vi "read_dust_control_settings_small.vi"(7 "Settings to be loaded":i32, 8 "error in (no error)":errorcluster, 9 "Tag Filter":cluster{"Tag":string, "Dust Type":string}, 10 "Lower Timestamp Range":timestamp, 11 "Upper Timestamp Range":timestamp) -> (0 "error out":errorcluster, 1 "Array":cluster{"String":string, "Value":dbl}[](array[cluster]), 3 "Dust Source Array":T1[](array[typedef]) {"Needle Voltage" min=0.0 max=10.0 step=0.01 format="%.2g"; "Desired Amplitude (V)" min=0.0 max=10.0 step=0.01 format="%5.2f"; "Width (ms) : 0.1" min=0.05 max=5.0 step=0.01 format="%6.2f"; "Frequency" min=1.0 max=100.0 step=0.01 format="%.1f"})   [LabVIEW 2013]
uses:
  dust_source_control_small.ctl
  <vilib>/addons/database/Auxilliary.llb/DB Tools Cursor Type.ctl
  <vilib>/addons/database/Connection.llb/Conn Execute.vi
  <vilib>/addons/database/Recordset.llb/Rec Fetch Recordset Data (R).vi
  <vilib>/addons/database/Recordset.llb/Rec Destroy - Connection.vi
  <vilib>/addons/database/_DB Variant To Data/Database Variant To Data.xnode
  <vilib>/addons/database/NI_Database_API.lvlib
panel:
  out "Settings ID 2":dbl(ring) caption="Settings ID" items=["Auto", "Auto", "Auto", "Auto", "Auto", "Auto", "Auto", "Auto", "Auto", "Auto", "Auto", "Auto", "Auto", "Auto", "Auto", "Auto", "Auto", "Auto", "Auto", "Auto", "Auto test", "Auto", "Automatic Update at  10/19/2012 4:35:52 PM", "Automatic Update at  10/19/2012 4:37:24 PM", "Automatic Update at  10/19/2012 4:37:56 PM", "Automatic Update at  10/19/2012 4:39:59 PM", "Automatic Update at  10/19/2012 4:40:46 PM", "Automatic Update at  10/19/2012 4:43:56 PM", "Automatic Update at  10/19/2012 5:03:34 PM", "Awesome settings that work", "Awesome settings that work", "Automatic Update at  10/19/2012 5:32:08 PM", "Automatic Update at  10/19/2012 5:34:15 PM", "Automatic Update at  10/19/2012 5:39:51 PM", "Working settings", "Working settings", "Working settings", "Working settings", "Working settings", "Automatic Update at  10/22/2012 1:18:52 PM", "Automatic Update at  10/22/2012 1:22:32 PM", "", "Test", "Test", "Automatic Update at  10/22/2012 1:29:56 PM", "Test", "Test 1", "Test 1", "Anna's Settings", "Automatic Update at  10/22/2012 3:57:19 PM", "test of width", "Automatic Update at  10/22/2012 4:02:00 PM", "Automatic Update at  10/22/2012 4:10:30 PM", "Automatic Update at  10/22/2012 4:15:00 PM", "Automatic Update at  10/22/2012 4:38:33 PM", "Automatic Update at  10/22/2012 4:44:48 PM", "Automatic Update at  10/22/2012 4:46:11 PM", "Automatic Update at  10/22/2012 4:51:36 PM", "Automatic Update at  10/22/2012 4:54:36 PM", "Automatic Update at  10/22/2012 4:59:09 PM", "Automatic Update at  10/22/2012 5:01:02 PM", "Automatic Update at  10/22/2012 5:06:29 PM", "Automatic Update at  10/22/2012 5:13:46 PM", "Automatic Update at  10/22/2012 5:18:54 PM", "Automatic Update at  10/22/2012 5:27:58 PM", "Automatic Update at  10/22/2012 5:37:45 PM", "Automatic Update at  10/22/2012 5:39:44 PM", "Automatic Update at  10/22/2012 5:41:21 PM", "Automatic Update at  10/22/2012 5:41:55 PM", "Automatic Update at  10/22/2012 5:43:41 PM", "Automatic Update at  10/22/2012 5:45:31 PM", "Anna's Settings (Updated with working Giraffes)", "Anna's Settings (Updated with working Giraffes)", "Automatic Update at  10/23/2012 1:01:38 PM", "test", "test", "test 1", "test 1", "Automatic Update at  10/23/2012 1:44:56 PM", "Automatic Update at  10/23/2012 1:52:29 PM", "Automatic Update at  10/23/2012 1:59:24 PM", "test 3", "test 4", "Automatic Update at  10/23/2012 2:20:20 PM", "Automatic Update at  10/23/2012 5:53:49 PM", "Anna's Settings", "Anna's Settings1", "test mctesty", "test mctesty", "Automatic Update at  10/24/2012 3:47:44 PM", "Test\"", "Test\"", "this is a \"test\" setting", "Automatic Update at  10/24/2012 4:13:56 PM"]
  out "SQL Query Sintax":string
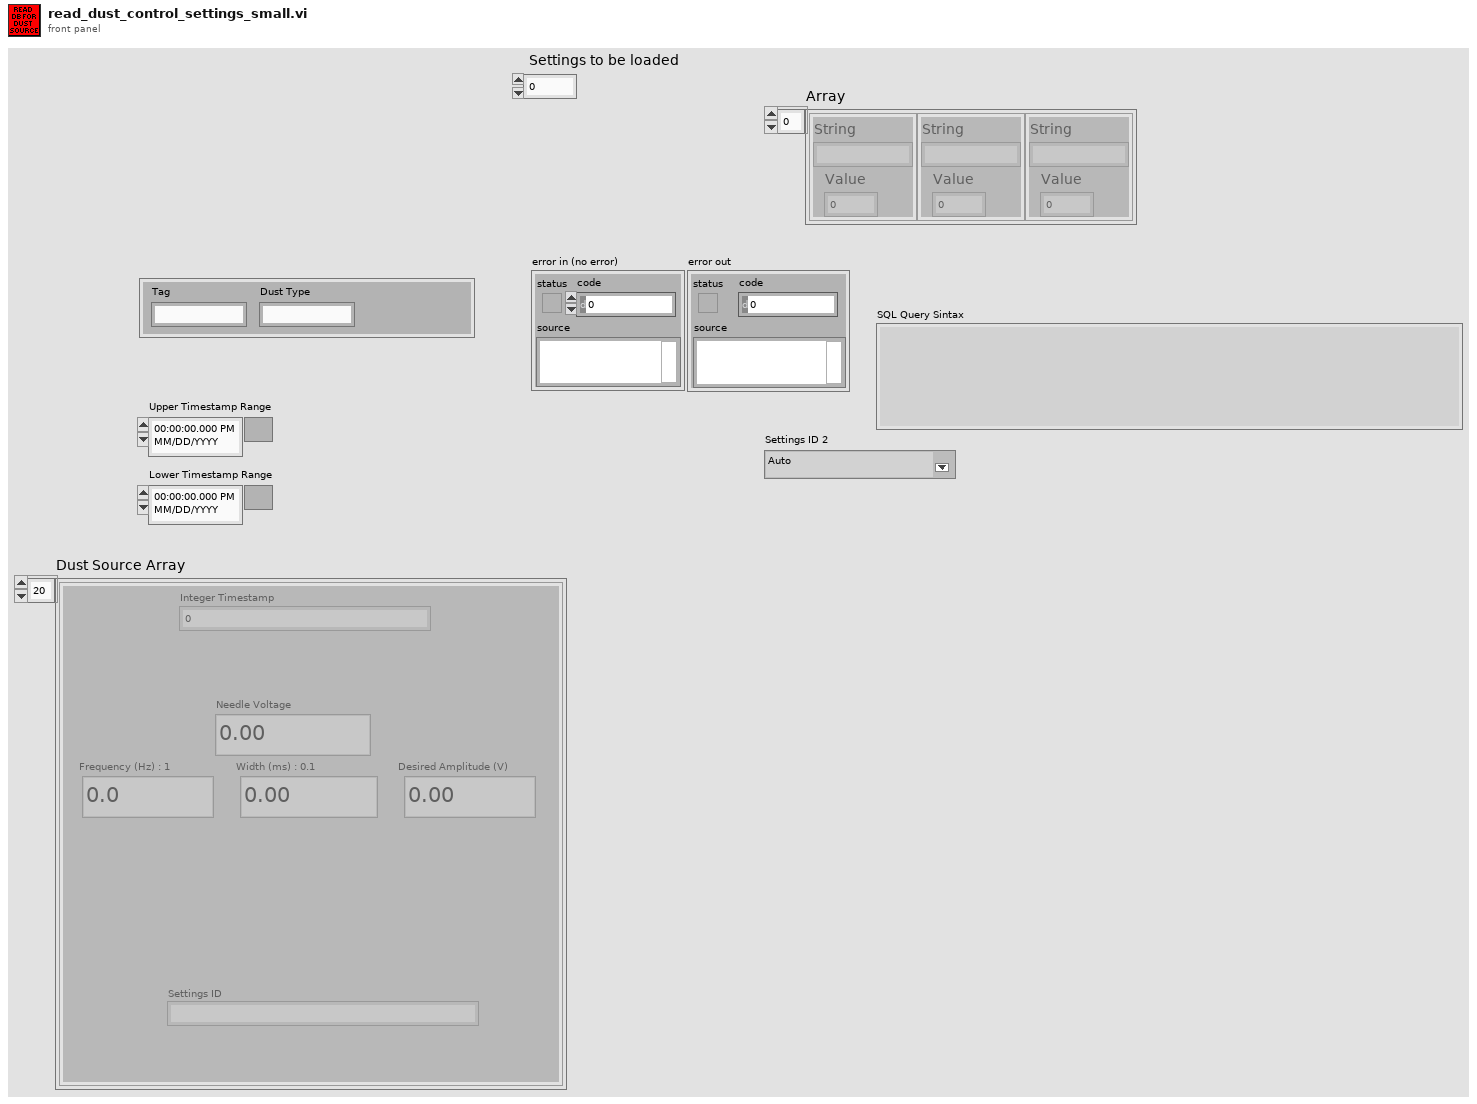
[diagram p1: front panel]
types:
  T1 = typedef "dust_source_control_small.ctl" = cluster{"Integer Timestamp":u64, "Needle Voltage":dbl, "Frequency":dbl, "Width (ms) : 0.1 ":dbl, "Desired Amplitude (V)":dbl, "Settings ID":string, "ID#":i32}
  T2 = typedef "NI_Database_API.lvlib/DB Tools Cursor Type.ctl" = enum16{"forward-only", "keyset", "dynamic", "static"}
  T3 = typedef "NI_Database_API.lvlib/Conn ObjectReference.ctl" = refnum<k1>
  T4 = typedef "NI_Database_API.lvlib/Rec ObjectReference.ctl" = refnum<k1>
  T5 = cluster{"Integer Timestamp":u64, "Needle Voltage":dbl, "Frequency":dbl, "Width (ms) : 0.1 ":dbl, "Desired Amplitude (V)":dbl, "Settings ID":string, "ID#":i32}
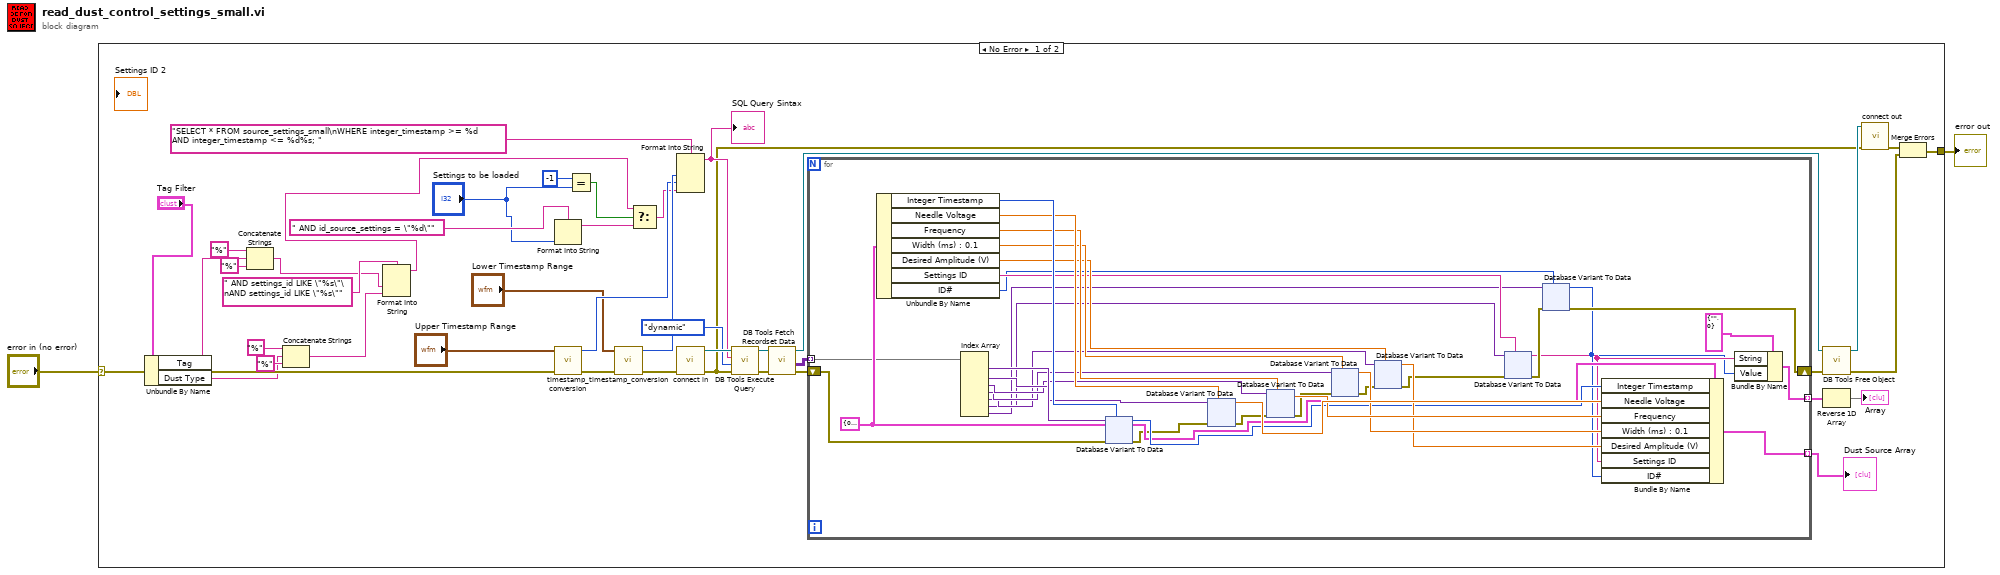
[diagram p0: block diagram]
diagram:
  n1 = case shown="No Error" "error in (no error)" {
    selector: "error in (no error)" -> [w35 w303]
    tunnel: [w19 w303] -> w1
    frame No Error {
      n2 = Unbundle By Name("Tag Filter") -> ("Tag"=w9:string, "Dust Type"=w7:string)
      n3 = Concatenate Strings("%" ("string"), w9, "%" ("string")) -> (w10:string)
      n4 = Concatenate Strings("%" ("string"), w7, "%" ("string")) -> (w5:string)
      n5 = Format Into String(format string=" AND settings_id LIKE \"%s\"\nAND settings_id LIKE \"%s\"" ("string"), w10, w5) -> (resulting string=w4:string)  [unwired: 2 in, 1 out]
      n6 = Format Into String(format string=" AND id_source_settings = \"%d\"" ("string"), "Settings to be loaded") -> (resulting string=w31:string)  [unwired: 2 in, 1 out]
      n7 = call "timestamp_conversion.vi"("error in (no error)"=w35, "Time Stamp"="Upper Timestamp Range") -> ("error out"=w36:errorcluster, "Integer Time"=w29:i64)  [unwired: 7 in]
      n8 = Equal?(x=-1, y="Settings to be loaded") -> (x = y?=w37:bool)
      n9 = call "timestamp_conversion.vi"("error in (no error)"=w36, "Time Stamp"="Lower Timestamp Range") -> ("error out"=w33:errorcluster, "Integer Time"=w30:i64)  [unwired: 7 in]
      n10 = Select(t=w4, s=w37, f=w31) -> (s? t:f=w23:string)
      n11 = Format Into String(format string="SELECT * FROM source_settings_small\nWHERE integer_timestamp >= %d  AND integer_timestamp <= %d%s; " ("string"), w30, w29, w23) -> (resulting string=w27:string)  [unwired: 2 in, 1 out]
      "SQL Query Sintax" <- w27
      n12 = call "connect in.vi"("error in (no error)"=w33) -> ("error out"=w17:errorcluster, "Database Connection"=w39:T3)  [unwired: 6 in, 1 out]
      n13 = call-poly <vilib>:"DB Tools Execute Query.vi"("error in (no error)"=w17, "cursor type"=DB_Tools_Cursor_Type."dynamic", "SQL query"=w27, "connection reference"=w39) -> ("error out"=w43:errorcluster, "recordset reference"=w44:T4)  [unwired: 4 in]
      n14 = call-poly <vilib>:"DB Tools Fetch Recordset Data.vi"("error in (no error)"=w43, "recordset reference"=w44) -> ("error out"=w41:errorcluster, "recordset data"=w34:variant[][], "recordset reference out"=w42:T4)  [unwired: 3 in]
      n15 = for {
        tunnel: w34 -> [w67] mode=indexing
        shift-right: [w58] -> w40
        shift-left: w41 -> [w78]
        tunnel: [w70] -> w14 mode=indexing
        tunnel: [w55] -> w22 mode=indexing
        w68 = T5 {"Integer Timestamp"=0, "Needle Voltage"=0.0, "Frequency"=1.0, "Width (ms) : 0.1 "=0.05, "Desired Amplitude (V)"=0.0, "Settings ID"="", "ID#"=0} ("Dust Source Controls")
        n16 = Unbundle By Name(w68) -> ("Integer Timestamp"=w66:u64, "Needle Voltage"=w64:dbl, "Frequency"=w63:dbl, "Width (ms) : 0.1"=w62:dbl, "Desired Amplitude (V)"=w61:dbl, "Settings ID"=w60:string, "ID#"=w57:i32)
        n17 = Index Array(array=w67) -> (element #1=w65:variant, element #2=w50:variant, element #3=w49:variant, element #4=w48:variant, element #5=w47:variant, element #6=w46:variant, element #7=w45:variant)  [unwired: 7 in]
        n18 = xnode "Database Variant To Data"("database variant"=w65, "error in"=w78, "type"=w66) -> ("data"=w69:u64, "error out"=w52:errorcluster)
        n19 = xnode "Database Variant To Data"("database variant"=w50, "error in"=w52, "type"=w64) -> ("data"=w77:dbl, "error out"=w75:errorcluster)
        n20 = xnode "Database Variant To Data"("database variant"=w49, "error in"=w75, "type"=w63) -> ("data"=w76:dbl, "error out"=w73:errorcluster)
        n21 = xnode "Database Variant To Data"("database variant"=w48, "error in"=w73, "type"=w62) -> ("data"=w74:dbl, "error out"=w72:errorcluster)
        n22 = xnode "Database Variant To Data"("database variant"=w47, "error in"=w72, "type"=w61) -> ("data"=w71:dbl, "error out"=w51:errorcluster)
        n23 = xnode "Database Variant To Data"("database variant"=w46, "error in"=w51, "type"=w60) -> ("data"=w54:string, "error out"=w59:errorcluster)
        n24 = xnode "Database Variant To Data"("database variant"=w45, "error in (no error)"=w59, "type"=w57) -> ("data"=w53:i32, "error out"=w58:errorcluster)
        n25 = Bundle By Name(cluster=w68, "Integer Timestamp"=w69, "Needle Voltage"=w77, "Frequency"=w76, "Width (ms) : 0.1"=w74, "Desired Amplitude (V)"=w71, "Settings ID"=w54, "ID#"=w53) -> (w70:T5)
        n26 = Bundle By Name(cluster=cluster{"String":string, "Value":i32} {"String"="", "Value"=0}, "String"=w54, "Value"=w53) -> (w55:cluster{"String":string, "Value":i32})
      }
      "Dust Source Array" <- w14
      n27 = call-poly <vilib>:"DB Tools Free Object.vi"("error in (no error)"=w40, "recordset reference"=w42) -> ("error out"=w18:errorcluster, "connection reference"=w38:T3)  [unwired: 8 in]
      n28 = Reverse 1D Array(array=w22) -> (reversed array=→"Array":cluster{"String":string, "Value":i32}[])
      n29 = call "connect out.vi"("error in (no error)"=w17, "connection reference"=w38) -> ("error out"=w20:errorcluster)  [unwired: 9 in]
      n30 = Merge Errors(w20, w18) -> (w19:errorcluster)
    }
    frame Error {
    }
  }
  "error out" <- w1
